vi "getXY.vi"(0 "数据":dbl[][](array[numeric]), 5 "传感器索引":i32, 7 "是否需要计算拟合曲线":bool) -> (3 "绝对偏差（mV）":dbl[](array[numeric]), 4 "x":dbl[](array[numeric]), 6 "y":dbl[](array[numeric]), 8 "预测期望值":dbl[](array[numeric]), 10 "拟合曲线":string, 13 "slope":dbl caption="斜率", 14 "intercept":dbl caption="截距", 15 "最大误差率":string)   [LabVIEW 2017]
uses:
  <vilib>/Analysis/6fits.llb/Curve Fitting Criteria.ctl
  <vilib>/Analysis/NI_AALPro.lvlib
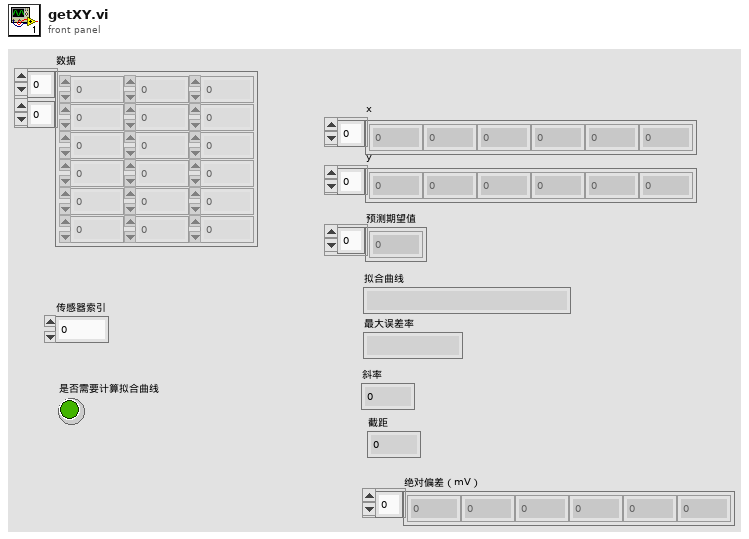
[diagram p1: front panel]
types:
  T1 = typedef "NI_AALPro.lvlib/Curve Fitting Criteria.ctl" = u16
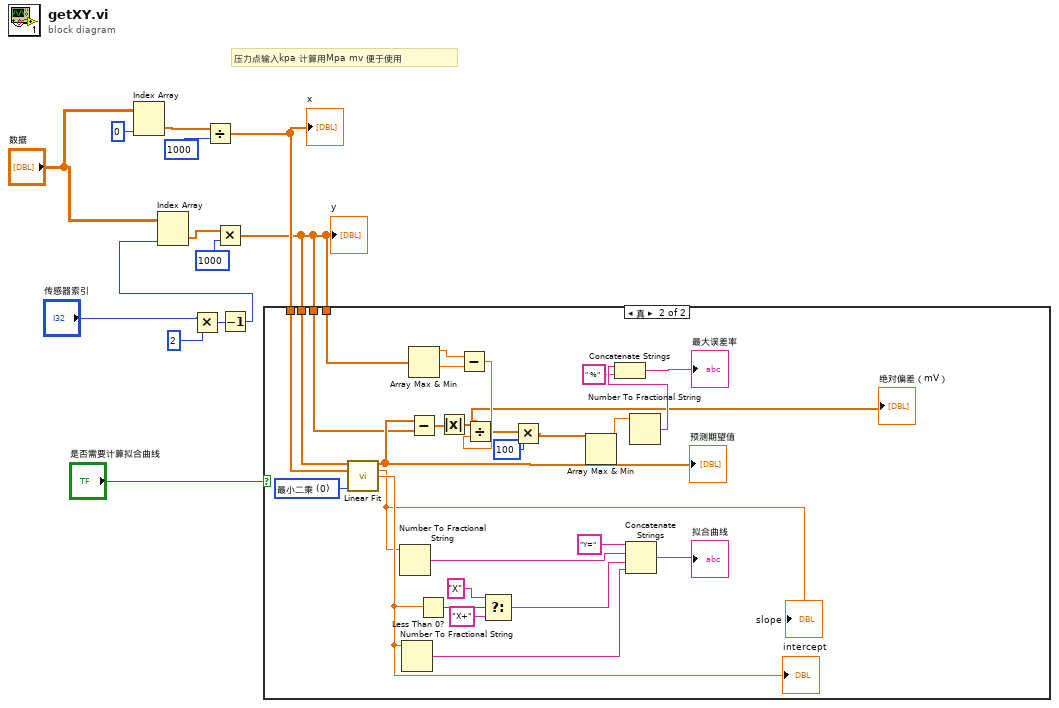
[diagram p0: block diagram]
diagram:
  # "压力点输入kpa 计算用Mpa mv 便于使用"
  n1 = Index Array(array="数据", index (col)=0 ("禁用的索引 (列)")) -> (element=w6:dbl[])  [unwired: 1 in]
  n2 = Multiply(x="传感器索引", y=2) -> (x*y=w12:i32)
  n3 = Divide(x=w6, y=1000) -> (x/y=w5:dbl[])
  "x" <- w5
  n4 = Decrement(x=w12) -> (x-1=w7:i32)
  n5 = Index Array(array="数据", index (col)=w7) -> (element=w3:dbl[])  [unwired: 1 in]
  n6 = Multiply(x=w3, y=1000) -> (x*y=w1:dbl[])
  "y" <- w1
  n7 = case shown="真" "是否需要计算拟合曲线" {
    tunnel: w5 -> [_ w31]
    tunnel: w1 -> [_ w30]
    tunnel: w1 -> [_ w28]
    tunnel: w1 -> [_ w27]
    frame False {
    }
    frame True {
      w32 = T1 0 items=["最小二乘", "最小绝对残差", "Bisquare"] ("method")
      n8 = call <vilib>:"Linear Fit.vi"("Y"=w30, "X"=w31, "method"=w32) -> ("Best Linear Fit"=w29:dbl[], "slope"=w36:dbl, "intercept"=w39:dbl)  [unwired: 8 in, 2 out]
      "预测期望值" <- w29
      "slope" <- w36
      "intercept" <- w39
      n9 = Number To Fractional String(number=w36) -> (F-format string=w37:string)  [unwired: 3 in]
      n10 = Number To Fractional String(number=w39) -> (F-format string=w41:string)  [unwired: 3 in]
      n11 = Array Max & Min(array=w27) -> (max value=w26:dbl, min value=w25:dbl)  [unwired: 2 out]
      n12 = Subtract(x=w29, y=w28) -> (x-y=w15:dbl[])
      n13 = Less Than 0?(x=w39) -> (x < 0?=w38:bool)
      n14 = Absolute Value(x=w15) -> (abs(x)=w14:dbl[])
      "绝对偏差（mV）" <- w14
      n15 = Subtract(x=w26, y=w25) -> (x-y=w24:dbl)
      n16 = Divide(x=w14, y=w24) -> (x/y=w22:dbl[])
      n17 = Select(t="X", s=w38, f="X+") -> (s? t:f=w40:string)
      n18 = Multiply(x=w22, y=100) -> (x*y=w16:dbl[])
      n19 = Array Max & Min(array=w16) -> (max value=w20:dbl)  [unwired: 3 out]
      n20 = Concatenate Strings("Y=" ("字符串"), w37, w40, w41) -> (→"拟合曲线":string)
      n21 = Number To Fractional String(number=w20) -> (F-format string=w19:string)  [unwired: 3 in]
      n22 = Concatenate Strings(w19, " %" ("字符串")) -> (→"最大误差率":string)
    }
  }
